vi "Launch MainTop.vi"   [LabVIEW 2021, in "Launcher.lvlib"]
uses:
  Launcher.lvlib
  UI_Top_Customer.lvclass
  C:/Program Files (x86)/National Instruments/LabVIEW 2021/vi.lib/ActorFramework/Actor/Actor.lvclass
  <vilib>/ActorFramework/Actor/Actor.lvclass
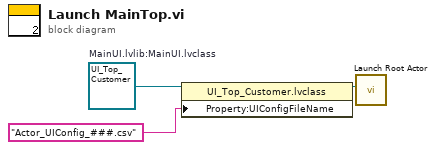
[diagram p0: block diagram]
diagram:
  w3 = refnum<class "UI_Top_Customer.lvclass"> refnum  # MainUI.lvlib:MainUI.lvclass
  n1 = property class="UI_Top_Customer.lvclass"(reference=w3, "Property:UIConfigFileName"="Actor_UIConfig_###.csv" ("UI: UIConfigFileName")) -> (reference out=w2:refnum<class "UI_Top_Customer.lvclass">)  [unwired: 1 in, 1 out]
  n2 = call <vilib>:"Launch Root Actor.vi"("Actor"=w2) -> ()  [unwired: 9 in, 2 out]
